vi "CloseDevice.vi"(8 "错误输入（无错误）":errorcluster, 10 "DevInd":u32, 11 "DeviceType":T1=3 items=["PCI-CAN200"=7, "USB-CAN"=2, "USB-CAN200"=3]) -> (0 "错误输出":errorcluster, 1 "DeviceInd":u32, 2 "Result":bool, 3 "DeviceTypeOut":T1=3 items=["PCI-CAN200"=7, "USB-CAN"=2, "USB-CAN200"=3])   [LabVIEW 2013]
uses:
  DevType.ctl
  VCI_CAN.dll
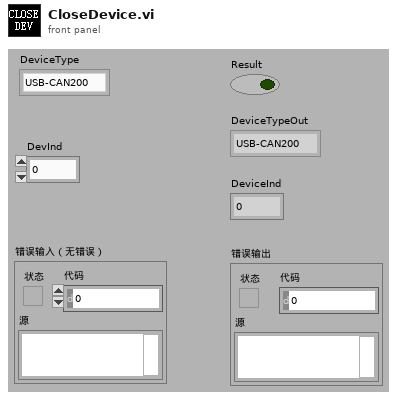
[diagram p1: front panel]
types:
  T1 = typedef "DevType.ctl" = u16
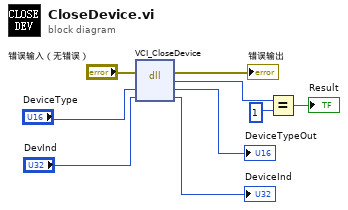
[diagram p0: block diagram]
diagram:
  n1 = dll-call lib="C:/Users/Administrator/Desktop/CAN/USBCAN/VCI_CAN.dll" fn="VCI_CloseDevice"(error in="错误输入（无错误）", "DeviceType"="DeviceType", "DeviceInd"="DevInd") -> (error out=→"错误输出":errorcluster, "返回类型"=w6:u32, "DeviceType"=→"DeviceTypeOut":u32, "DeviceInd"=→"DeviceInd":u32)  [unwired: 2 in, 1 out]
  n2 = Equal?(x=w6, y=u32 1) -> (x = y?=→"Result":bool)
